vi "SpectralBiclustering.vi"(8 "error in":errorcluster) -> (0 "error out":errorcluster, 3 "out":refnum<class "SpectralBiclustering.lvclass">)   [LabVIEW 2020]
doc: "Spectral biclustering (Kluger, 2003).\n\n Partitions rows and columns under the assumption that the data has\n an underlying checkerboard structure. For instance, if there are\n two row partitions and three column partitions, each row will\n belong to three biclusters, and each column will belong to two\n biclusters. The outer product of the corresponding row and column\n label vectors gives this checkerboard structure.\n\n Read more in the :ref:`User Guide <spectral_biclustering>`.\n\n Parameters\n ----------\n n_clusters : int or tuple (n_row_clusters, n_column_clusters), default=3\n The number of row and column clusters in the checkerboard\n structure.\n\n method : {'bistochastic', 'scale', 'log'}, default='bistochastic'\n Method of normalizing and converting singular vectors into\n biclusters. May be one of 'scale', 'bistochastic', or 'log'.\n The authors recommend using 'log'. If the data is sparse,\n however, log normalization will not work, which is why the\n default is 'bistochastic'.\n\n .. warning::\n if `method='log'`, the data must be sparse.\n\n n_components : int, default=6\n Number of singular vectors to check.\n\n n_best : int, default=3\n Number of best singular vectors to which to project the data\n for clustering.\n\n svd_method : {'randomized', 'arpack'}, default='randomized'\n Selects the algorithm for finding singular vectors. May be\n 'randomized' or 'arpack'. If 'randomized', uses\n :func:`~sklearn.utils.extmath.randomized_svd`, which may be faster\n for large matrices. If 'arpack', uses\n `scipy.sparse.linalg.svds`, which is more accurate, but\n possibly slower in some cases.\n\n n_svd_vecs : int, default=None\n Number of vectors to use in calculating the SVD. Corresponds\n to `ncv` when `svd_method=arpack` and `n_oversamples` when\n `svd_method` is 'randomized`.\n\n mini_batch : bool, default=False\n Whether to use mini-batch k-means, which is faster but may get\n different results.\n\n init : {'k-means++', 'random'} or ndarray of (n_clusters, n_features), default='k-means++'\n Method for initialization of k-means algorithm; defaults to\n 'k-means++'.\n\n n_init : int, default=10\n Number of random initializations that are tried with the\n k-means algorithm.\n\n If mini-batch k-means is used, the best initialization is\n chosen and the algorithm runs once. Otherwise, the algorithm\n is run for each initialization and the best solution chosen.\n\n n_jobs : int, default=None\n The number of jobs to use for the computation. This works by breaking\n down the pairwise matrix into n_jobs even slices and computing them in\n parallel.\n\n ``None`` means 1 unless in a :obj:`joblib.parallel_backend` context.\n ``-1`` means using all processors. See :term:`Glossary <n_jobs>`\n for more details.\n\n .. deprecated:: 0.23\n ``n_jobs`` was deprecated in version 0.23 and will be removed in\n 1.0 (renaming of 0.25).\n\n random_state : int, RandomState instance, default=None\n Used for randomizing the singular value decomposition and the k-means\n initialization. Use an int to make the randomness deterministic.\n See :term:`Glossary <random_state>`.\n\n Attributes\n ----------\n rows_ : array-like of shape (n_row_clusters, n_rows)\n Results of the clustering. `rows[i, r]` is True if\n cluster `i` contains row `r`. Available only after calling ``fit``.\n\n columns_ : array-like of shape (n_column_clusters, n_columns)\n Results of the clustering, like `rows`.\n\n row_labels_ : array-like of shape (n_rows,)\n Row partition labels.\n\n column_labels_ : array-like of shape (n_cols,)\n Column partition labels.\n\n \nAvailable methods:\nGet Attributes\nGet Params\nSet Params"
uses:
  SpectralBiclustering.lvclass
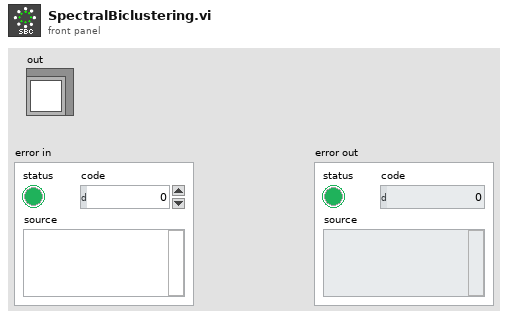
[diagram p1: front panel]
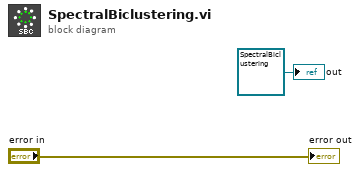
[diagram p0: block diagram]
diagram:
  "out" <- refnum<class "SpectralBiclustering.lvclass"> refnum ("model")
  "error out" <- "error in"
